vi "Mesure-distance-par-reflexion-optique.vi"() -> ()   [LabVIEW 2019]
uses:
  <vilib>/Instr/_visa.llb/VISA Configure Serial Port (Instr).vi
panel:
  in  "Démarrer":bool
  in  "Arrêt":bool
  in  "VISA resource name":refnum<visa-resource-name> caption="Nom de ressource VISA"
  out "Graphe déroulant":i32(graph)
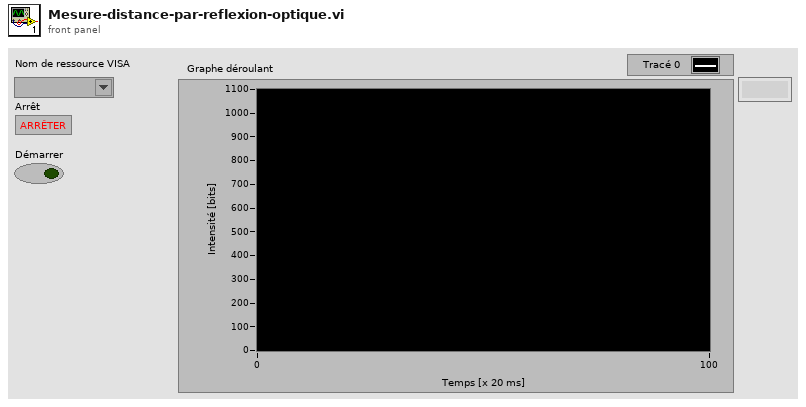
[diagram p1: front panel]
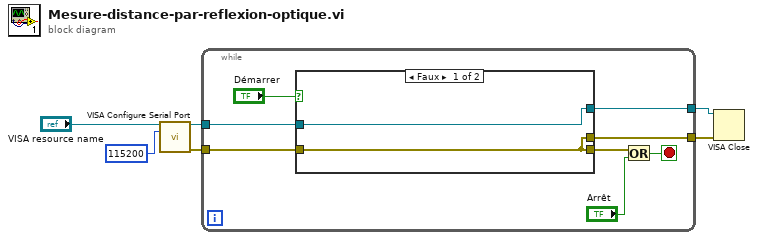
[diagram p0: block diagram]
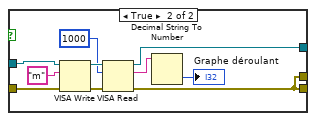
[diagram p2: hidden frame]
diagram:
  n1 = call-poly "VISA Configure Serial Port"("VISA resource name"="VISA resource name", "baud rate (9600)"=u32 115200) -> ("VISA resource name out"=w4:refnum<visa-resource-name>, "error out"=w3:errorcluster)  [unwired: 12 in]
  n2 = while {
    tunnel: w4 -> [w13]
    tunnel: w3 -> [w12]
    tunnel: [w8] -> w2
    tunnel: [w7] -> w1
    stop <- w9 stop-if-true
    n3 = case shown="Faux" "Démarrer" {
      tunnel: w13 -> [w16 w26]
      tunnel: w12 -> [w15 w25]
      tunnel: [w15 w17] -> w10
      tunnel: [w16 w20] -> w8
      tunnel: [w15 w17] -> w7
      frame False {
      }
      frame True {
        n4 = VISA Write(VISA resource name=w26, write buffer="m" ("buffer d'écriture"), error in (no error)=w25) -> (VISA resource name out=w22:refnum<visa-resource-name>, error out=w24:errorcluster)  [unwired: 1 out]
        n5 = VISA Read(VISA resource name=w22, byte count=u32 1000 ("nombre d'octets"), error in (no error)=w24) -> (VISA resource name out=w20:refnum<visa-resource-name>, read buffer=w19:string, error out=w17:errorcluster)  [unwired: 1 out]
        n6 = Decimal String To Number(string=w19) -> (number=→"Graphe déroulant":i32)  [unwired: 2 in, 1 out]
      }
    }
    n7 = Or(x=w10, y="Arrêt") -> (x .or. y?=w9:bool)
  }
  n8 = VISA Close(VISA resource name=w2, error in (no error)=w1) -> ()  [unwired: 1 out]
